vi "Configure Flow Rate.vi"(5 "Retry Attempts (0)":i32 min=0, 7 "Fast Comms (F)":bool, 8 "error in":errorcluster, 10 "Flow Input (ml/min)":dbl, 11 "VISA resource name":refnum<visa-resource-name>) -> (0 "error out":errorcluster, 3 "VISA resource name out":refnum<visa-resource-name>)   [LabVIEW 2020, in "ChromTech Series I Drivers.lvlib"]
doc: "Configures the flow rate using up to 5 digits. If the entered value exceeds the maximum allowable flow rate of the pump, the flow rate will be automatically set to the maximum allowable flow rate. The maximum allowable flow rate can be found using the Get Maximum Flow Rate VI and the current flow rate can be found using the Get Current Flow Rate VI or Get Current Conditions VI"
uses:
  <instrlib>/RxnRover/ChromtechSeriesIDriver/ChromTech Series I Drivers.lvlib
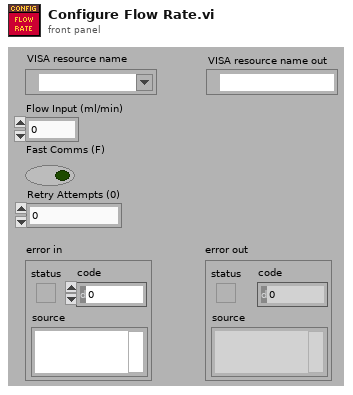
[diagram p1: front panel]
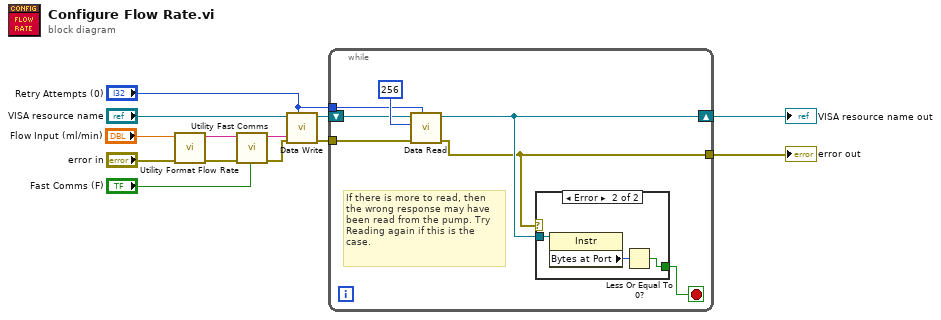
[diagram p0: block diagram]
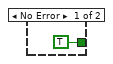
[diagram p2: hidden frame]
diagram:
  n1 = call <instrlib>:"Utility Format Flow Rate.vi"("error in (no error)"="error in", "Flow Rate"="Flow Input (ml/min)") -> ("error out"=w8:errorcluster, "Formatted Flow Rate"=w7:string)  [unwired: 8 in]
  n2 = call <instrlib>:"Utility Fast Comms.vi"("Fast Comms"="Fast Comms (F)", "Command"=w7) -> ("Fast Command"=w6:string)  [unwired: 9 in]
  n3 = call <instrlib>:"Data Write.vi"("Retry Attempts (0)"="Retry Attempts (0)", "error in (no error)"=w8, "Command"=w6, "VISA Refnum in"="VISA resource name") -> ("error out"=w11:errorcluster, "VISA Refnum out"=w4:refnum<visa-resource-name>)  [unwired: 6 in]
  n4 = while {
    tunnel: "Retry Attempts (0)" -> [w16]
    shift-right: [w15] -> w2
    shift-left: w4 -> [w17]
    tunnel: w11 -> [w19]
    tunnel: [w14] -> w1
    stop <- w13 stop-if-true
    # "If there is more to read, then\nthe wrong response may have\nbeen read from the pump. Try\nReading again if this is the\ncase."
    n5 = call <instrlib>:"Data Read.vi"("Retry Attempts (0)"=w16, "error in (no error)"=w19, "Bytes to read"=256, "VISA Refnum in"=w17) -> ("error out"=w14:errorcluster, "VISA Refnum out"=w15:refnum<visa-resource-name>)  [unwired: 5 in, 1 out]
    n6 = case shown="Error" w14 {
      tunnel: w15 -> [_ w23]
      tunnel: [TRUE w21] -> w13
      frame No Error {
      }
      frame Error {
        n7 = property class="Instr"(reference=w23) -> ("Bytes at Port"=w22:u32)  [unwired: 1 in, 2 out]
        n8 = Less Or Equal To 0?(x=w22) -> (x <= 0?=w21:bool)
      }
    }
  }
  "VISA resource name out" <- w2
  "error out" <- w1
